vi "Data_GetImage.vi"(8 "error in (no error)":errorcluster caption="错误输入（无错误）", 11 "Picture_Class 输入":refnum<class "Picture_Class.lvclass"> caption="DNL_LabVIEW Object in") -> (0 "error out":errorcluster caption="错误输出", 1 "image data":T1, 2 "Picture Out":picture, 3 "Picture_Class 输出":refnum<class "Picture_Class.lvclass"> caption="DNL_LabVIEW Object out")   [LabVIEW 2013, in "Picture_Class.lvclass"]
uses:
  Picture_Class.lvclass
  <vilib>/picture/picture.llb/imagedata.ctl
  Picture_Class.lvclass/Picture_Class.ctl
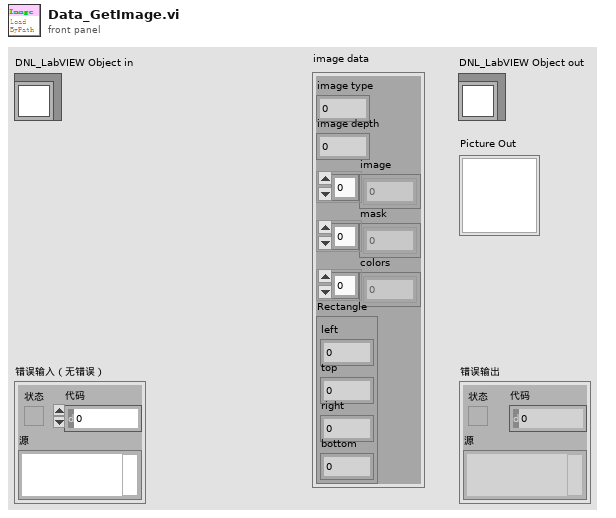
[diagram p1: front panel]
types:
  T1 = typedef "imagedata.ctl" = cluster{"image type":i32, "image depth":i32, "image":u8[], "mask":u8[], "colors":u32[], "Rectangle":cluster{"left":i16, "top":i16, "right":i16, "bottom":i16}}
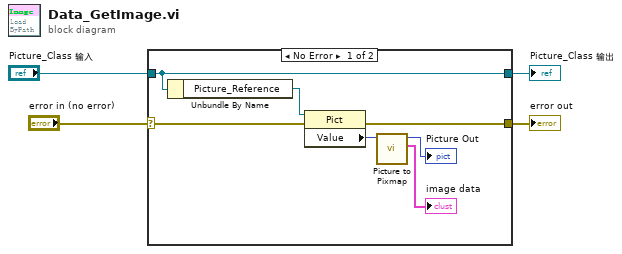
[diagram p0: block diagram]
diagram:
  n1 = case shown="No Error" "error in (no error)" {
    selector: "error in (no error)" -> [w9 w13]
    tunnel: [w10 w13] -> w3
    tunnel: [w11 w12] -> w1
    tunnel: "Picture_Class 输入" -> [w11 w12]
    frame No Error {
      n2 = Unbundle By Name(w11) -> ("Picture_Reference"=w8:refnum<vi>)
      n3 = property class="Pict"(reference=w8, error in=w9) -> (error out=w10:errorcluster, "Value"=w7:picture)  [unwired: 1 out]
      n4 = call <vilib>:"Picture to Pixmap.vi"("picture"=w7) -> ("image data"=→"image data":T1, "new picture"=→"Picture Out":picture)  [unwired: 9 in]
    }
    frame Error {
    }
  }
  "error out" <- w3
  "Picture_Class 输出" <- w1
